vi "Analyse_Pulse.vi"() -> ()   [LabVIEW 2024]
panel:
  in  "Array":path[](array[path])
  out "Waveform Graph 2":i16[][](graph)
  in  "Split count":i32=65536 format="0x%x (%d)"
  in  "channel name(s) in":string="in"
  in  "group name in":string="p"
  out "Waveform Graph":i16[][](graph)
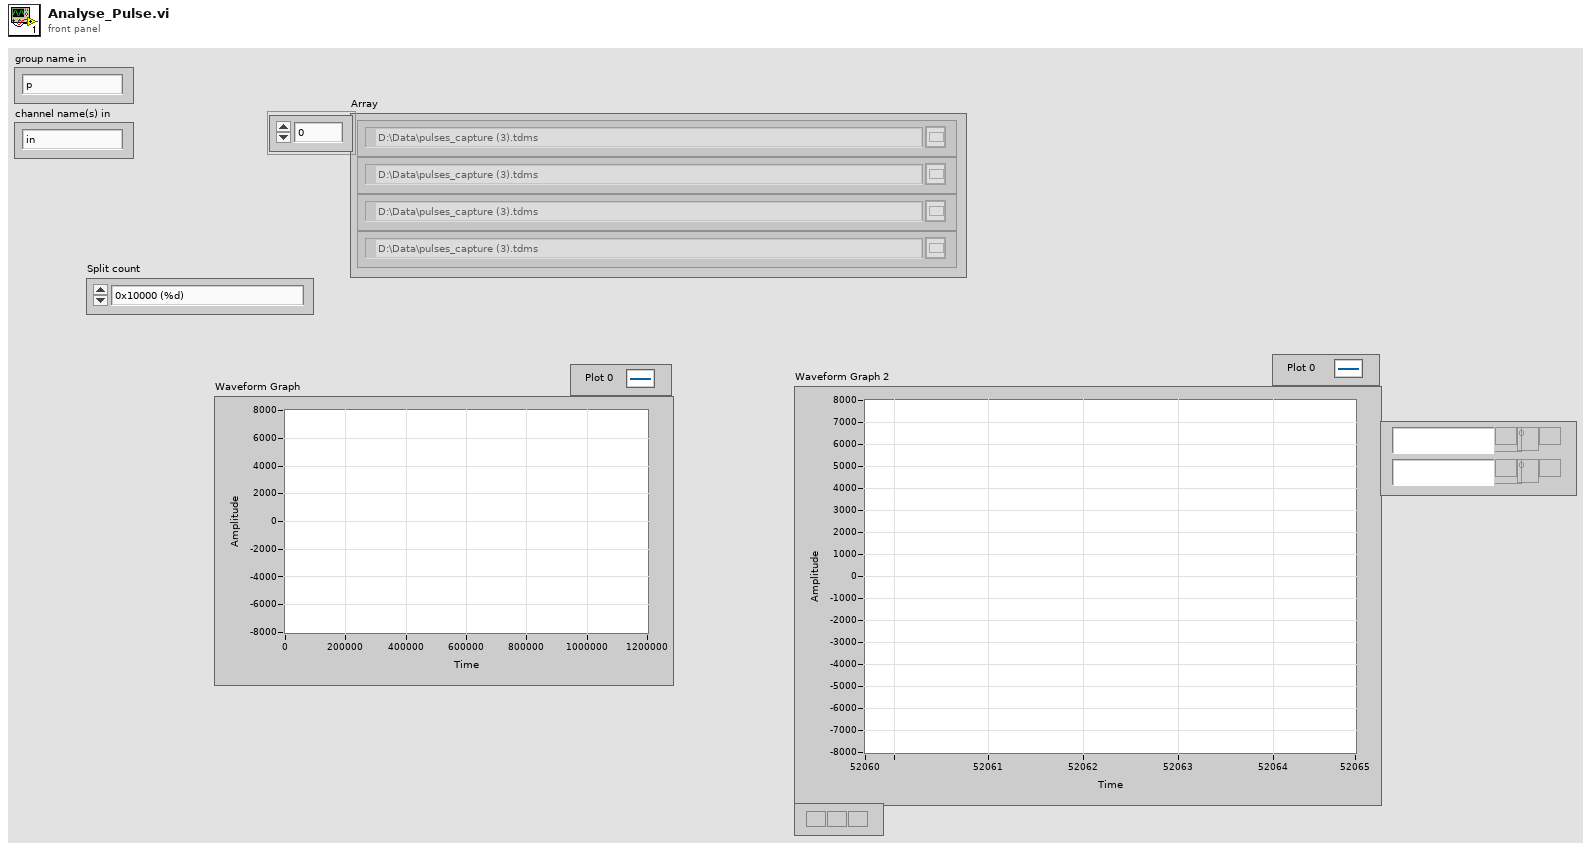
[diagram p1: front panel]
types:
  T1 = enum16{"open", "open or create", "create or replace", "create", "open (read-only)"}
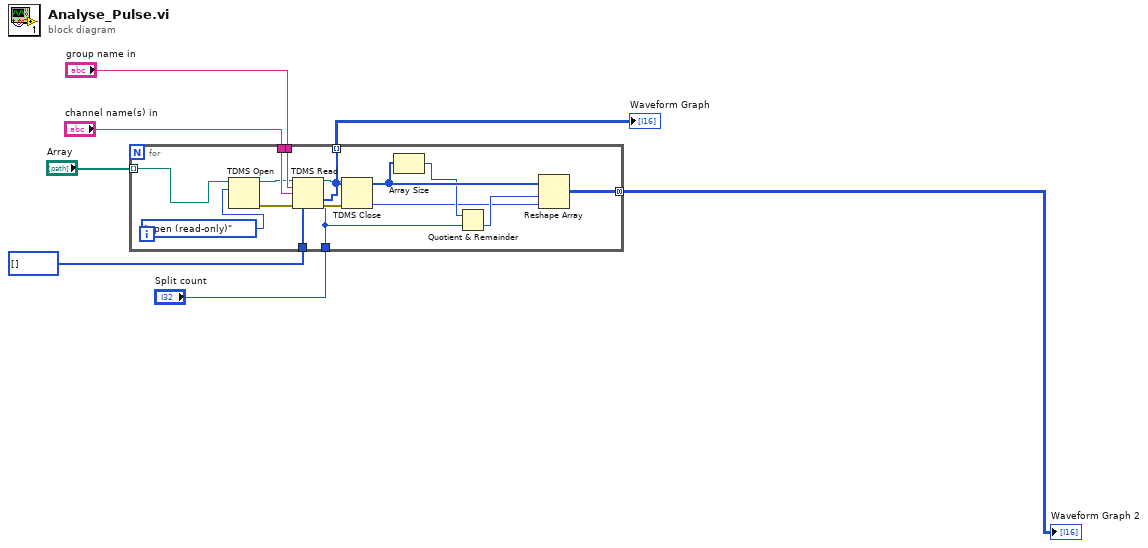
[diagram p0: block diagram]
diagram:
  n1 = for {
    tunnel: i16[] [] -> [w19]
    tunnel: "group name in" -> [w18]
    tunnel: "channel name(s) in" -> [w17]
    tunnel: [w13] -> w4 mode=concatenating
    tunnel: [w12] -> w3 mode=indexing
    tunnel: "Split count" -> [w9]
    tunnel: "Array" -> [w8] mode=indexing
    n2 = TDMS Open(10:T1."open (read-only)" ("operation (0:open)"), 11:w8) -> (0:w20:errorcluster, 3:w15:refnum<k34>)  [unwired: 5 in]
    n3 = TDMS Read(0:w15, 5:w18, 7:w17, 11:w20, 12:w19) -> (4:w14:refnum<k34>, 10:w12:i16[], 15:w16:errorcluster)  [unwired: 3 in, 3 out]
    n4 = TDMS Close(8:w16, 11:w14) -> ()  [unwired: 2 out]
    n5 = Array Size(array=w12) -> (size(s)=w11:i32)
    n6 = Quotient & Remainder(x=w11, y=w9) -> (floor(x/y)=w10:i32)  [unwired: 1 out]
    n7 = Reshape Array(w12, w10, w9) -> (w13:i16[][])
  }
  "Waveform Graph" <- w3
  "Waveform Graph 2" <- w4
